vi "Open TLCameraSDK.vi"(8 "error in (no error)":errorcluster) -> (0 "error out":errorcluster, 3 "TLCameraSDK ref out":refnum<k24>)   [LabVIEW 2020]
uses:
  C:/GEECS/Developers Version/builds/Device builds/ThorlabsCsCamera/Thorlabs.TSI.TLCameraInterfaces.dll
  Thorlabs.TSI.TLCameraInterfaces.dll
  C:/GEECS/Developers Version/builds/Device builds/ThorlabsCsCamera/Thorlabs.TSI.TLCamera.dll
  Thorlabs.TSI.TLCamera.dll
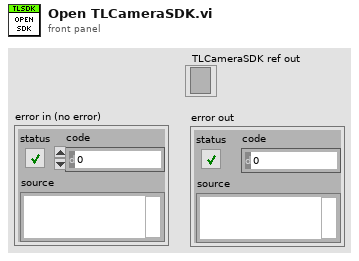
[diagram p1: front panel]
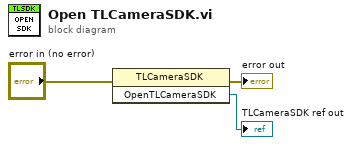
[diagram p0: block diagram]
diagram:
  n1 = invoke class="TLCameraSDK" method="OpenTLCameraSDK"(error in="error in (no error)") -> (error out=→"error out":errorcluster, "OpenTLCameraSDK"=→"TLCameraSDK ref out":refnum<k24>)  [unwired: 2 in, 1 out]
